vi "E03.vi"() -> ()   [LabVIEW 2020]
panel:
  out "n!/(n-r)!":dbl
  in  "r":i32
  in  "n":i32
  in  "Botón de paro":bool
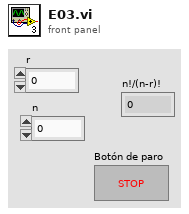
[diagram p1: front panel]
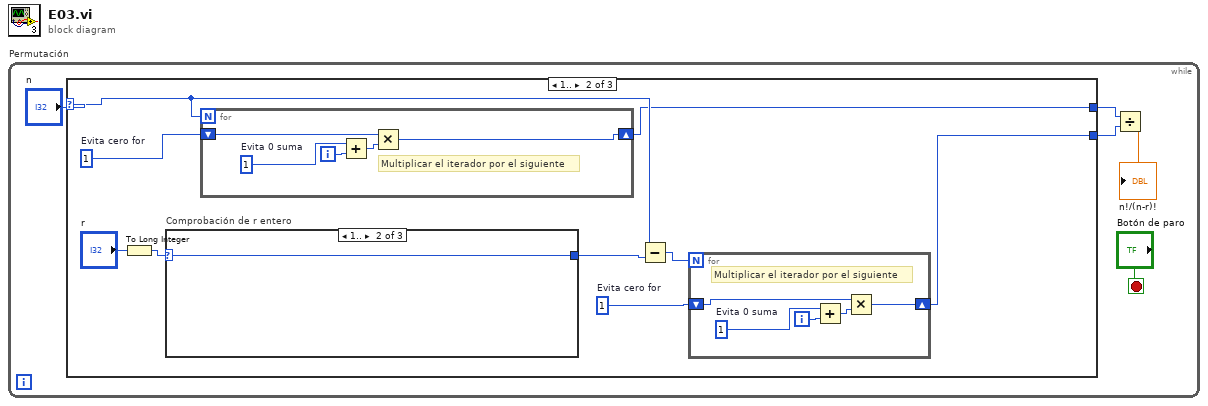
[diagram p0: block diagram]
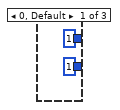
[diagram p2: hidden frame]
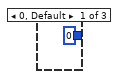
[diagram p3: hidden frame]
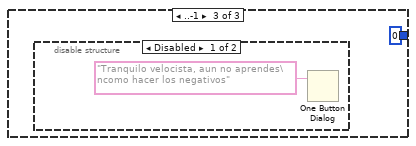
[diagram p4: hidden frame]
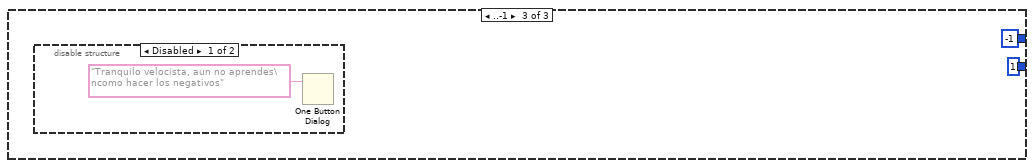
[diagram p6: hidden frame]
diagram:
  n1 = while "Permutación" {
    stop <- "Botón de paro" stop-if-true
    n2 = case shown="1.." "n" {
      selector: "n" -> [_ w14 _]
      tunnel: [1 w9 -1] -> w3
      tunnel: [1 ("Evita cero for") w8 1 ("Evita cero for")] -> w2
      frame 0, Default {
      }
      frame 1.. {
        w15 = 1  # Evita cero for
        w16 = 1  # Evita cero for
        n3 = To Long Integer(number="r") -> (32bit integer=w12:i32)
        n4 = case "Comprobación de r entero" shown="1.." w12 {
          selector: w12 -> [_ w18 _]
          tunnel: [0 w18 0] -> w11
          frame 0, Default {
          }
          frame 1.. {
          }
          frame ..-1 {
            n5 = disable-structure shown="Disabled" {
              frame Disabled {
                n6 = One Button Dialog(message="Tranquilo velocista, aun no aprendes\ncomo hacer los negativos") -> ()  [unwired: 1 in, 1 out]
              }
              frame Enabled {
              }
            }
          }
        }
        n7 = for {
          N: w14 -> [_]
          shift-right: [w29] -> w9
          shift-left: w16 -> [w30]
          i -> [w28]
          w26 = 1  # Evita 0 suma
          # "Multiplicar el iterador por el siguiente"
          n8 = Add(x=w26, y=w28) -> (x+y=w27:i32)
          n9 = Multiply(x=w30, y=w27) -> (x*y=w29:i32)
        }
        n10 = Subtract(x=w14, y=w11) -> (x-y=w10:i32)
        n11 = for {
          N: w10 -> [_]
          shift-right: [w24] -> w8
          shift-left: w15 -> [w25]
          i -> [w23]
          w21 = 1  # Evita 0 suma
          # "Multiplicar el iterador por el siguiente"
          n12 = Add(x=w21, y=w23) -> (x+y=w22:i32)
          n13 = Multiply(x=w25, y=w22) -> (x*y=w24:i32)
        }
      }
      frame ..-1 {
        n14 = disable-structure shown="Disabled" {
          frame Disabled {
            n15 = One Button Dialog(message="Tranquilo velocista, aun no aprendes\ncomo hacer los negativos") -> ()  [unwired: 1 in, 1 out]
          }
          frame Enabled {
          }
        }
      }
    }
    n16 = Divide(x=w3, y=w2) -> (x/y=→"n!/(n-r)!":dbl)
  }
